vi "New Command Packet.vi"(8 "error in (no error)":errorcluster, 11 "Command ID":u16) -> (0 "error out":errorcluster, 3 "Packet out":refnum<class "Packet.lvclass">)   [LabVIEW 2020, in "Communication Classes.lvlib" / "Packet.lvclass"]
uses:
  Packet.lvclass
  Packet.lvclass/Packet.ctl
  Accessors/Write Command ID.vi
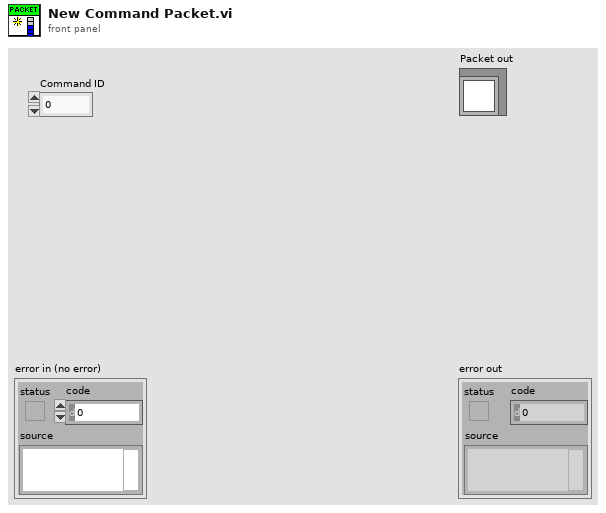
[diagram p1: front panel]
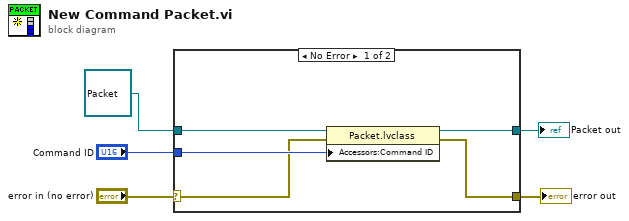
[diagram p0: block diagram]
diagram:
  n1 = case shown="No Error" "error in (no error)" {
    selector: "error in (no error)" -> [w9 w12]
    tunnel: [w8 w12] -> w4
    tunnel: "Command ID" -> [w10 _]
    tunnel: [w7 w11] -> w2
    tunnel: refnum<class "Packet.lvclass"> refnum ("Communication.lvlib:Packet.lvclass") -> [w6 w11]
    frame No Error {
      n2 = property class="Packet.lvclass"(reference=w6, error in=w9, "Accessors:Command ID"=w10) -> (reference out=w7:refnum<class "Packet.lvclass">, error out=w8:errorcluster)
    }
    frame Error {
    }
  }
  "error out" <- w4
  "Packet out" <- w2
